vi "onProcessStart.vi"(8 "error in (no error)":errorcluster, 11 "Subsystem":refnum<class "DAQmx(AI).lvclass">) -> (0 "error out":errorcluster, 3 "Subsystem out":refnum<class "DAQmx(AI).lvclass">)   [LabVIEW 2013, in "DAQmx(AI).lvclass"]
doc: "JKI State Machine Objects (SMO) 1.1.8.32\nJKI - JKI\nCopyright (c) 2016, JKI"
uses:
  DAQmx(AI).lvclass
  <vilib>/JKI/JKI SMO/SMO/SMO.lvclass
  <vilib>/DAQmx/create/channels.llb/DAQmx Create Channel (AI-Voltage-Basic).vi
  <vilib>/DAQmx/create/channels.llb/DAQmx Create Channel (AI-Current-Basic).vi
  <resource>/objmgr/daqmx.rc
panel:
  # "For instructions on how to use the JKI State Machine Objects, examples and video tutorials, visit:\nhttp://jki.net/state-machine-objects/\n\nJKI State Machine Objects™\nhttp://jki.net/state-machine-objects/\nCopyright (C) 2005-2015, JKI <info@jki.net>\nALL RIGHTS RESERVED"
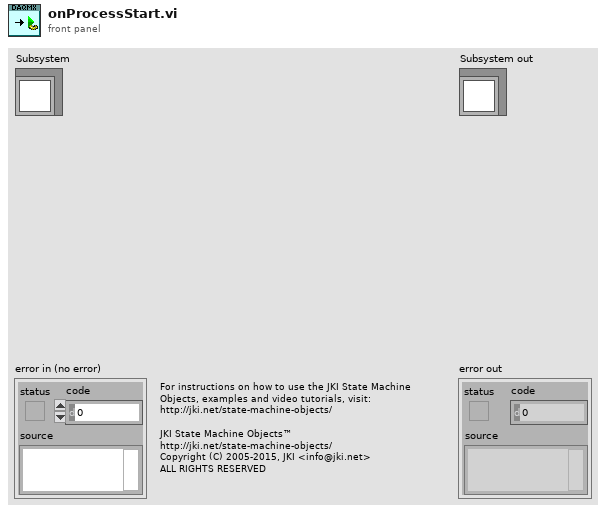
[diagram p1: front panel]
types:
  T1 = typedef "DAQmx(AI).lvclass/Configuration--Cluster.ctl" = cluster{"PhysChan":tag, "Period (ms)":i64, "input terminal cfg":i32, "minimum value":dbl, "maximum value":dbl, "units":T2, "task name":string}
  T2 = typedef "DAQmx(AI).lvclass/Units -- Enum.ctl" = enum16{"Volts", "Amps", "Deg F", "Deg C", "Deg R", "Kelvins", "Strain", "Ohms", "Hz", "Seconds", "Meters", "Inches", "Degrees", "Radians", "Ticks", "g", "m/s^2", "m/s", "in/s", "Pascals", "Newtons", "Pounds", "kgf", "psi", "bar", "Nm", "oz-in", "lb-in", "lb-ft", "Volts/Volt", "mVolts/Volt", "From TEDS"}
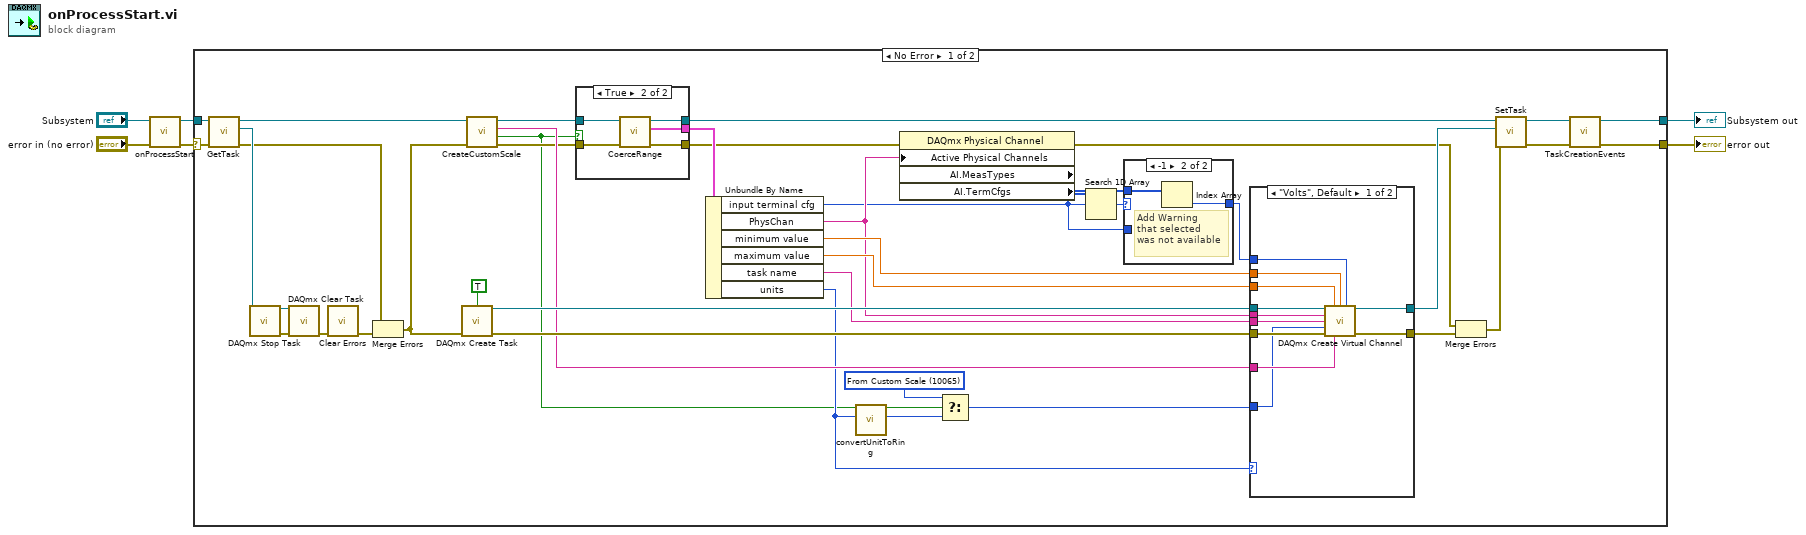
[diagram p0: block diagram]
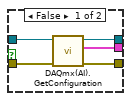
[diagram p3: hidden frame]
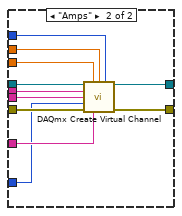
[diagram p4: hidden frame]
diagram:
  n1 = call-parent "onProcessStart.vi"("error in (no error)"="error in (no error)", "SMO"="Subsystem") -> ("error out"=w1:errorcluster, "SMO out"=w4:refnum<class "DAQmx(AI).lvclass">)  [unwired: 8 in]
  n2 = case shown="No Error" w1 {
    selector: w1 -> [w40 w83]
    tunnel: w4 -> [w41 w82]
    tunnel: [w7 w82] -> w3
    tunnel: [w8 w83] -> w2
    frame No Error {
      w22 = 10065 items=["Volts"=10348, "From Custom Scale"=10065] ("units")
      n3 = call "GetTask.vi"("error in (no error)"=w40, "Subsystem"=w41) -> ("error out"=w34:errorcluster, "task"=w37:refnum<k21>, "Subsystem out"=w26:refnum<class "DAQmx(AI).lvclass">)  [unwired: 7 in]
      n4 = call <vilib>:"DAQmx Stop Task.vi"("task/channels in"=w37) -> ("task out"=w38:refnum<k21>, "error out"=w39:errorcluster)  [unwired: 13 in]
      n5 = call <vilib>:"DAQmx Clear Task.vi"("task in"=w38, "error in"=w39) -> ("error out"=w36:errorcluster)  [unwired: 13 in]
      n6 = call <vilib>:"Clear Errors.vi"("error in (no error)"=w36) -> ("error out"=w35:errorcluster)  [unwired: 6 in]
      n7 = Merge Errors(w34, w35) -> (w25:errorcluster)
      n8 = call <vilib>:"DAQmx Create Task.vi"("auto cleanup"=TRUE, "error in"=w25) -> ("task out"=w46:refnum<k21>, "error out"=w45:errorcluster)  [unwired: 12 in]
      n9 = call "CreateCustomScale.vi"("error in (no error)"=w25, "Subsystem in"=w26) -> ("error out"=w17:errorcluster, "Custom Scaling"=w16:bool, "Custom Scale"=w24:tag, "Subsystem out"=w18:refnum<class "DAQmx(AI).lvclass">)  [unwired: 6 in]
      n10 = case shown="True" w16 {
        tunnel: [w50 w55] -> w44
        tunnel: [w51 w59] -> w19
        tunnel: [w52 w58] -> w13
        tunnel: w18 -> [w54 w57]
        tunnel: w17 -> [w53 w56]
        frame False {
          n11 = call "DAQmx(AI).GetConfiguration.vi"("error in (no error)"=w53, "Subsystem"=w54) -> ("error out"=w52:errorcluster, "Configuration"=w50:T1, "Subsystem out"=w51:refnum<class "DAQmx(AI).lvclass">)  [unwired: 7 in]
        }
        frame True {
          n12 = call "CoerceRange.vi"("error in (no error)"=w56, "DAQmx(AI) in"=w57) -> ("error out"=w58:errorcluster, "Configuration"=w55:T1, "DAQmx(AI) out"=w59:refnum<class "DAQmx(AI).lvclass">)  [unwired: 7 in]
        }
      }
      n13 = Unbundle By Name(w44) -> ("input terminal cfg"=w9:i32, "PhysChan"=w15:tag, "minimum value"=w29:dbl, "maximum value"=w28:dbl, "task name"=w27:string, "units"=w23:T2)
      n14 = call "convertUnitToRing.vi"("Units"=w23) -> ("DAQmx units (Ring)"=w21:i32)  [unwired: 10 in]
      n15 = property class="DAQmx Physical Channel" props=["Active Physical Channels", "AI.MeasTypes", "AI.TermCfgs"](error in=w13, "Active Physical Channels"=w15) -> (error out=w14:errorcluster, "AI.TermCfgs"=w11:i32[])  [unwired: 1 in, 2 out]
      n16 = Select(t=w22, s=w16, f=w21) -> (s? t:f=w20:i32)
      n17 = Search 1D Array(1D array=w11, element=w9) -> (index of element=w12:i32)  [unwired: 1 in]
      n18 = case shown="-1" w12 {
        tunnel: w11 -> [_ w49]
        tunnel: [w47 w48] -> w10
        tunnel: w9 -> [w47 _]
        frame Default {
        }
        frame -1 {
          # "Add Warning\nthat selected\nwas not available"
          n19 = Index Array(array=w49) -> (element=w48:i32)  [unwired: 1 in]
        }
      }
      n20 = case shown="\"Volts\", Default" w23 {
        tunnel: w46 -> [w70 w81]
        tunnel: w45 -> [w69 w80]
        tunnel: w15 -> [w68 w79]
        tunnel: [w67 w78] -> w42
        tunnel: [w66 w77] -> w32
        tunnel: w10 -> [w65 w76]
        tunnel: w29 -> [w64 w75]
        tunnel: w28 -> [w63 w74]
        tunnel: w27 -> [w62 w73]
        tunnel: w24 -> [w61 w72]
        tunnel: w20 -> [w60 w71]
        frame "Volts", Default {
          n21 = call-poly <vilib>:"DAQmx Create Virtual Channel.vi"("task in"=w70, "maximum value"=w63, "minimum value"=w64, "input terminal configuration"=w65, "physical channels"=w68, "name to assign"=w62, "units"=w60, "error in"=w69, "custom scale name"=w61) -> ("task out"=w66:refnum<k21>, "error out"=w67:errorcluster)  [unwired: 5 in]
        }
        frame "Amps" {
          n22 = call-poly <vilib>:"DAQmx Create Virtual Channel.vi"("task in"=w81, "maximum value"=w74, "minimum value"=w75, "input terminal configuration"=w76, "physical channels"=w79, "name to assign"=w73, "units"=w71, "error in"=w80, "custom scale name"=w72) -> ("task out"=w77:refnum<k21>, "error out"=w78:errorcluster)  [unwired: 5 in]
        }
      }
      n23 = Merge Errors(w14, w42) -> (w33:errorcluster)
      n24 = call "SetTask.vi"("error in (no error)"=w33, "task"=w32, "Subsystem"=w19) -> ("error out"=w30:errorcluster, "Subsystem out"=w31:refnum<class "DAQmx(AI).lvclass">)  [unwired: 7 in]
      n25 = call "TaskCreationEvents.vi"("error in (no error)"=w30, "DAQmx(AI) in"=w31) -> ("error out"=w8:errorcluster, "DAQmx(AI) out"=w7:refnum<class "DAQmx(AI).lvclass">)  [unwired: 8 in]
    }
    frame Error {
    }
  }
  "error out" <- w2
  "Subsystem out" <- w3
